vi "Milk dispense control.vi"() -> ()   [LabVIEW 2019]
panel:
  in  "milliseconds to wait":u32
  in  "MD_R":bool
  in  "MD_L":bool
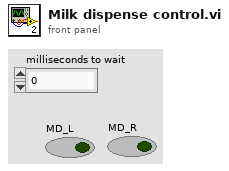
[diagram p1: front panel]
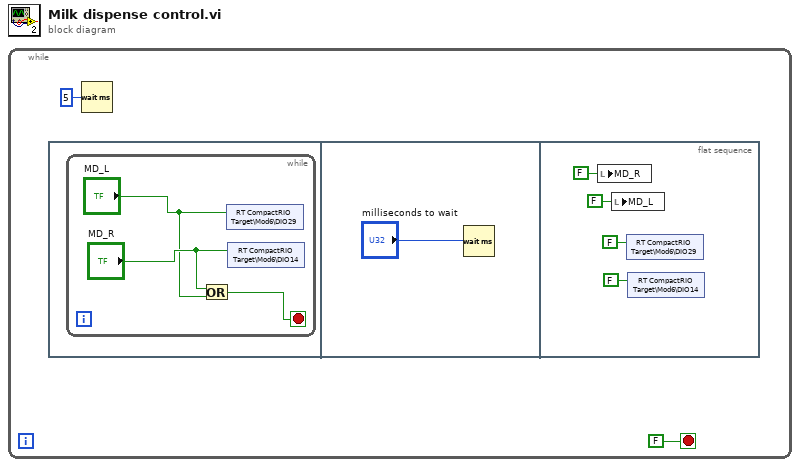
[diagram p0: block diagram]
diagram:
  n1 = while {
    stop <- FALSE stop-if-true
    n2 = flat-sequence {
      frame #0 {
        n3 = while {
          stop <- w3 stop-if-true
          n4 = Or(x="MD_R", y="MD_L") -> (x .or. y?=w3:bool)
          n5 = shared-variable "RT CompactRIO Target\\Mod6\\DIO29"("MD_L") -> ()  [unwired: 1 in, 1 out]
          n6 = shared-variable "RT CompactRIO Target\\Mod6\\DIO14"("MD_R") -> ()  [unwired: 1 in, 1 out]
        }
      }
      frame #1 {
        n7 = Wait (ms)(milliseconds to wait="milliseconds to wait") -> ()  [unwired: 1 out]
      }
      frame #2 {
        n8 = local write "MD_R"(FALSE ("MD_R")) -> ()
        n9 = local write "MD_L"(FALSE ("MD_L")) -> ()
        n10 = shared-variable "RT CompactRIO Target\\Mod6\\DIO29"(FALSE ("DIO29")) -> ()  [unwired: 1 in, 1 out]
        n11 = shared-variable "RT CompactRIO Target\\Mod6\\DIO14"(FALSE ("DIO14")) -> ()  [unwired: 1 in, 1 out]
      }
    }
    n12 = Wait (ms)(milliseconds to wait=u32 5) -> ()  [unwired: 1 out]
  }
